vi "DataLogger_OpenFile.vi"(6 "base path (C:\\CAlex\\)":path=path "C:/CAlex", 7 "File Extension (txt)":string="txt", 8 "error in (no error)":errorcluster, 9 "Header":string, 10 "File Name":string, 11 "Data Logger in":refnum<class "Data Logger.lvclass">) -> (0 "error out":errorcluster, 3 "Data Logger out":refnum<class "Data Logger.lvclass">)   [LabVIEW 2016, in "Data Logger.lvclass"]
uses:
  Data Logger.lvclass
  Data Logger.lvclass/Data Logger.ctl
panel:
  # "."
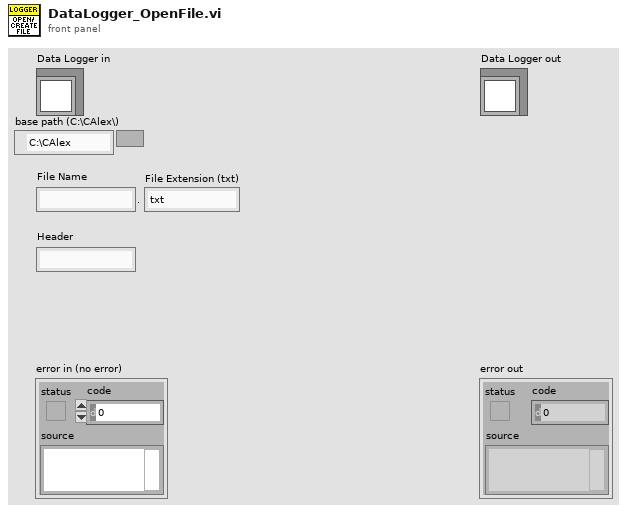
[diagram p1: front panel]
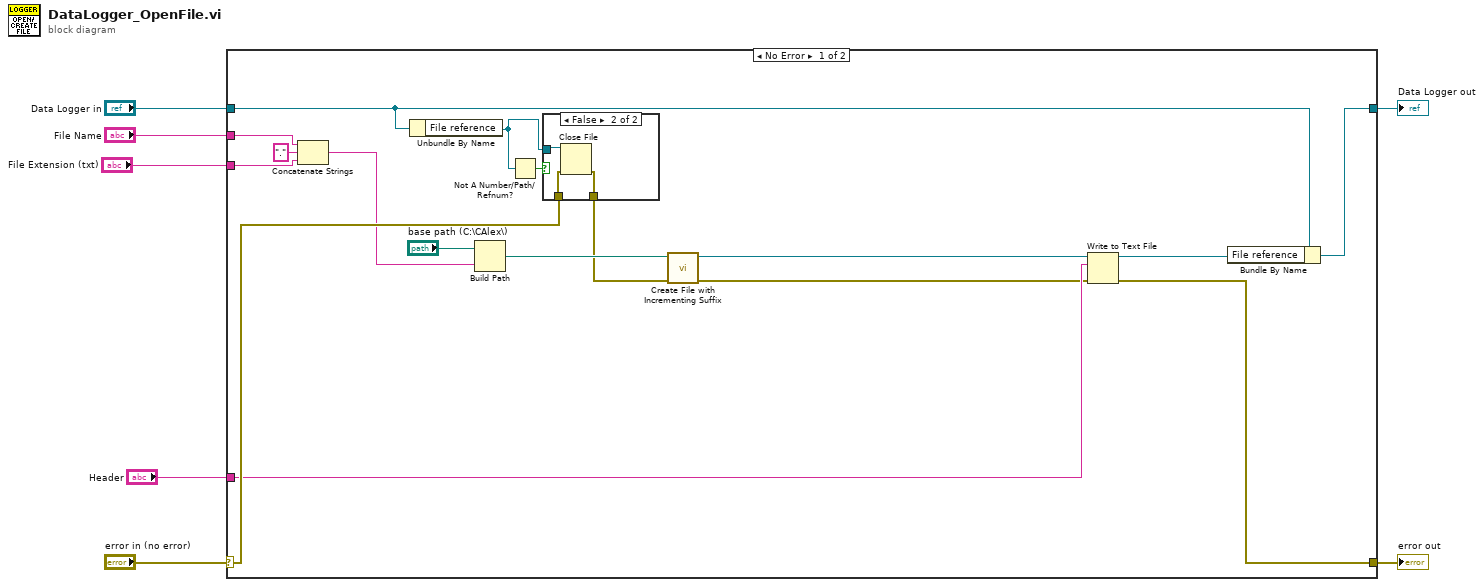
[diagram p0: block diagram]
diagram:
  n1 = case shown="No Error" "error in (no error)" {
    selector: "error in (no error)" -> [w22 w30]
    tunnel: [w21 w30] -> w6
    tunnel: [w23 w29] -> w4
    tunnel: "Data Logger in" -> [w24 w29]
    tunnel: "File Name" -> [w9 _]
    tunnel: "Header" -> [w20 _]
    tunnel: "File Extension (txt)" -> [w10 _]
    frame No Error {
      n2 = Concatenate Strings(w9, "." ("string"), w10) -> (w19:string)
      n3 = Unbundle By Name(w24) -> ("File reference"=w13:refnum<file>)
      n4 = Build Path(base path="base path (C:\\CAlex\\)", name or relative path=w19) -> (appended path=w16:path)
      n5 = Not A Number/Path/Refnum?(number/path/refnum=w13) -> (NaN/Path/Refnum?=w14:bool)
      n6 = case shown="False" w14 {
        tunnel: w13 -> [_ w28]
        tunnel: w22 -> [w25 w27]
        tunnel: [w25 w26] -> w15
        frame True {
        }
        frame False {
          n7 = Close File(refnum=w28, error in=w27) -> (error out=w26:errorcluster)  [unwired: 1 out]
        }
      }
      n8 = call <vilib>:"Create File with Incrementing Suffix.vi"("error in (no error)"=w15, "file path"=w16) -> ("error out"=w11:errorcluster, "refnum out"=w12:refnum<file>)  [unwired: 7 in, 1 out]
      n9 = Write to Text File(file (use dialog)=w12, text=w20, error in=w11) -> (refnum out=w17:refnum<file>, error out=w21:errorcluster)  [unwired: 1 in, 1 out]
      n10 = Bundle By Name(cluster=w24, "File reference"=w17) -> (w23:refnum<class "Data Logger.lvclass">)
    }
    frame Error {
    }
  }
  "error out" <- w6
  "Data Logger out" <- w4
